vi "Power_Meter_Switch(S5).vi"(8 "error in":errorcluster, 10 "Output":T1(ring)=enum."Power Meter (J6)", 11 "Input":T2(ring)=enum."Signal Source Switch (S4)") -> (0 "error out":errorcluster, 2 "Verfied":bool, 3 "Switches":string)   [LabVIEW 2012]
panel:
  # "Power Meter Switch (S5)"
  # "Switch Output"
  # "Switch Input"
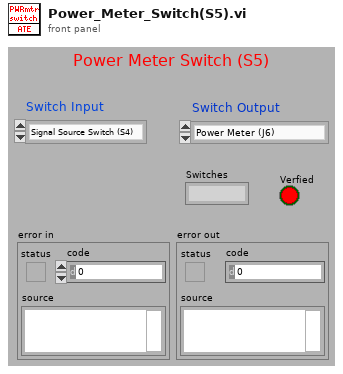
[diagram p1: front panel]
types:
  T1 = enum16{"NONE", "Power Meter (J6)", "IO Switch # 1", "IO Switch # 2"}
  T2 = enum16{"NONE", "IO Switch #1 (S1)", "Signal Source Switch (S4)", "Signal Out Switch (S3)", "IO Switch #2 (S2)", "TXH-TXV Switch (J8)"}
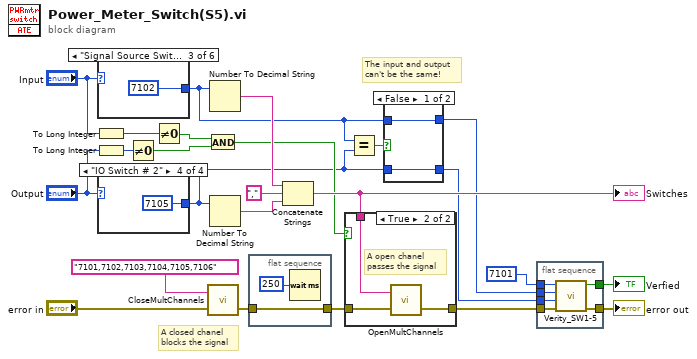
[diagram p0: block diagram]
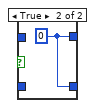
[diagram p2: hidden frame]
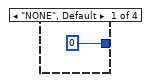
[diagram p3: hidden frame]
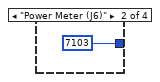
[diagram p4: hidden frame]
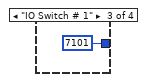
[diagram p5: hidden frame]
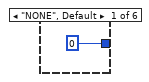
[diagram p6: hidden frame]
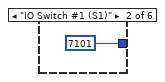
[diagram p7: hidden frame]
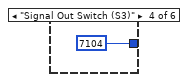
[diagram p8: hidden frame]
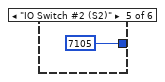
[diagram p9: hidden frame]
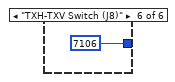
[diagram p10: hidden frame]
diagram:
  # "The input and output\ncan't be the same!"
  # "A closed chanel\nblocks the signal"
  n1 = To Long Integer(number="Input") -> (32bit integer=w13:i32)
  n2 = To Long Integer(number="Output") -> (32bit integer=w14:i32)
  n3 = case shown="\"Signal Source Switch (S4)\"" "Input" {
    tunnel: [0 7101 7102 7104 7105 7106] -> w3
    frame "NONE", Default {
    }
    frame "IO Switch #1 (S1)" {
    }
    frame "Signal Source Switch (S4)" {
    }
    frame "Signal Out Switch (S3)" {
    }
    frame "IO Switch #2 (S2)" {
    }
    frame "TXH-TXV Switch (J8)" {
    }
  }
  n4 = case shown="\"IO Switch # 2\"" "Output" {
    tunnel: [0 7103 7101 7105] -> w2
    frame "NONE", Default {
    }
    frame "Power Meter (J6)" {
    }
    frame "IO Switch # 1" {
    }
    frame "IO Switch # 2" {
    }
  }
  n5 = Not Equal To 0?(x=w14) -> (x != 0?=w15:bool)
  n6 = Not Equal To 0?(x=w13) -> (x != 0?=w16:bool)
  n7 = And(x=w16, y=w15) -> (x .and. y?=w10:bool)
  n8 = call "CloseMultChannels.vi"("error in (no error)"="error in", "Channels to be closed"="7101,7102,7103,7104,7105,7106" ("Channels to be opened")) -> ("error out"=w22:errorcluster)  [unwired: 1 in]
  n9 = Number To Decimal String(number=w3) -> (decimal integer string=w20:string)  [unwired: 1 in]
  n10 = Number To Decimal String(number=w2) -> (decimal integer string=w19:string)  [unwired: 1 in]
  n11 = flat-sequence {
    tunnel: w22 -> [w35]
    tunnel: [w35] -> w21
    frame #0 {
      n12 = Wait (ms)(milliseconds to wait=u32 250) -> ()  [unwired: 1 out]
    }
  }
  n13 = Concatenate Strings(w20, ",", w19) -> (w17:string)
  "Switches" <- w17
  n14 = case shown="True" w10 {
    tunnel: w21 -> [w37 w39]
    tunnel: w17 -> [_ w40]
    tunnel: [w37 w38] -> w8
    frame False {
    }
    frame True {
      # "A open chanel\npasses the signal"
      n15 = call "OpenMultChannels.vi"("error in (no error)"=w39, "Channels to be opened"=w40) -> ("error out"=w38:errorcluster)  [unwired: 1 in]
    }
  }
  n16 = Equal?(x=w3, y=w2) -> (x = y?=w6:bool)
  n17 = case shown="False" w6 {
    tunnel: w2 -> [w41 _]
    tunnel: [w41 w43] -> w5
    tunnel: w3 -> [w42 _]
    tunnel: [w42 w43] -> w4
    frame False {
    }
    frame True {
      w43 = 0 ("Switch ID")
    }
  }
  n18 = flat-sequence {
    tunnel: 7101 ("Switch ID") -> [w49]
    tunnel: w4 -> [w48]
    tunnel: w5 -> [w47]
    tunnel: [w46] -> w9
    tunnel: w8 -> [w45]
    tunnel: [w44] -> w7
    frame #0 {
      n19 = call "Verity_SW1-5.vi"("error in"=w45, "Output Switch ID"=w47, "Input Switch ID"=w48, "Base Switch ID"=w49) -> ("error out"=w44:errorcluster, "Verfied"=w46:bool)  [unwired: 6 in]
    }
  }
  "error out" <- w7
  "Verfied" <- w9
